vi "Activate Menu.vi"(8 "error in (no error)":errorcluster, 9 "Run mode?":bool, 10 "MenuRef":refnum<k9>, 11 "2D Plot.lvclass in":refnum<class "2D Plot.lvclass">) -> (0 "error out":errorcluster, 3 "2D Plot.lvclass out":refnum<class "2D Plot.lvclass">)   [LabVIEW 2017, in "2D Plot.lvclass"]
uses:
  <vilib>/Math Plots/2D Math Plots/2D Plot/2D Plot/2D Plot.lvclass
  <vilib>/Math Plots/2D Math Plots/2D Plot/2D Plot/2D Plot.lvclass/2D Plot.ctl
panel:
  in  "New Item Names":string="Auto Size Plot Legend"
  in  "Run-time Menu":T1(array[cluster])=[{"menu tag"="", "items to delete"=["APP_SC_CLEAR_GRAPH", "APP_SC_AUTOSCALE_X", "APP_SC_AUTOSCALE_Y", "APP_SC_SMOOTH_UPDATES", "APP_SC_OPTIONAL_PLANE", "APP_SC_SHOW_DIAGRAM"], "new menu"=[{"item names"="Clear Graph", "item tags"="USER_SC_CLEAR_GRAPH", "after item"="APP_SC_CLEAR_GRAPH"}, {"item names"="Autoscale X", "item tags"="USER_SC_AUTOSCALE_X", "after item"="APP_SC_AUTOSCALE_X"}, {"item names"="Autoscale Y", "item tags"="USER_SC_AUTOSCALE_Y", "after item"="USER_SC_AUTOSCALE_X"}], "root?"=TRUE}, {"menu tag"="APP_SC_VISIBLE_ITEMS", "items to delete"=["APP_SC_PLOT_LEGEND", "APP_SC_SCALE_LEGEND", "APP_SC_GRAPH_PALETTE", "APP_SC_CURSOR_LEGEND", "APP_SC_X_SCROLLBAR", "APP_SC_X_SCALE", "APP_SC_Y_SCALE", "APP_SC_UNIT_LABEL"], "new menu"=[{"item names"="Plot Legend", "item tags"="USER_SC_PLOT_LEGEND", "after item"="APP_SC_SEPERATOR"}, {"item names"="Scale Legend", "item tags"="USER_SC_SCALE_LEGEND", "after item"="USER_SC_PLOT_LEGEND"}, {"item names"="Graph Palette", "item tags"="USER_SC_GRAPH_PALETTE", "after item"="USER_SC_SCALE_LEGEND"}, {"item names"="Cursor Legend", "item tags"="USER_SC_CURSOR_LEGEND", "after item"="USER_SC_GRAPH_PALETTE"}, {"item names"="X Scrollbar", "item tags"="USER_SC_X_SCROLLBAR", "after item"="USER_SC_CURSOR_LEGEND"}, {"item names"="-", "item tags"="APP_SC_SEPERATOR", "after item"="USER_SC_X_SCROLLBAR"}, {"item names"="X Scale", "item tags"="USER_SC_X_SCALE", "after item"="APP_SC_SEPERATOR"}, {"item names"="Y Scale", "item tags"="USER_SC_Y_SCALE", "after item"="USER_SC_X_SCALE"}], "root?"=FALSE}]
  in  "Edit-time Menu":T1(array[cluster])=[{"menu tag"="", "items to delete"=["APP_SC_AUTOSCALE_X", "APP_SC_AUTOSCALE_Y", "APP_SC_SMOOTH_UPDATES", "APP_SC_OPTIONAL_PLANE", "APP_SC_PROPERTIES"], "new menu"=[{"item names"="Autoscale X", "item tags"="USER_SC_AUTOSCALE_X", "after item"="APP_SC_AUTOSCALE_X"}, {"item names"="Autoscale Y", "item tags"="USER_SC_AUTOSCALE_Y", "after item"="USER_SC_AUTOSCALE_X"}, {"item names"="Properties", "item tags"="USER_SC_PROPERTIES", "after item"="APP_SC_SEPARATOR"}], "root?"=TRUE}, {"menu tag"="APP_SC_VISIBLE_ITEMS", "items to delete"=["APP_SC_PLOT_LEGEND", "APP_SC_SCALE_LEGEND", "APP_SC_GRAPH_PALETTE", "APP_SC_CURSOR_LEGEND", "APP_SC_X_SCROLLBAR", "APP_SC_X_SCALE", "APP_SC_Y_SCALE", "APP_SC_UNIT_LABEL"], "new menu"=[{"item names"="Plot Legend", "item tags"="USER_SC_PLOT_LEGEND", "after item"="APP_SC_SEPERATOR"}, {"item names"="Scale Legend", "item tags"="USER_SC_SCALE_LEGEND", "after item"="USER_SC_PLOT_LEGEND"}, {"item names"="Graph Palette", "item tags"="USER_SC_GRAPH_PALETTE", "after item"="USER_SC_SCALE_LEGEND"}, {"item names"="Cursor Legend", "item tags"="USER_SC_CURSOR_LEGEND", "after item"="USER_SC_GRAPH_PALETTE"}, {"item names"="X Scrollbar", "item tags"="USER_SC_X_SCROLLBAR", "after item"="USER_SC_CURSOR_LEGEND"}, {"item names"="-", "item tags"="APP_SC_SEPERATOR", "after item"="USER_SC_X_SCROLLBAR"}, {"item names"="X Scale", "item tags"="USER_SC_X_SCALE", "after item"="APP_SC_SEPERATOR"}, {"item names"="Y Scale", "item tags"="USER_SC_Y_SCALE", "after item"="USER_SC_X_SCALE"}], "root?"=FALSE}, {"menu tag"="APP_SC_ADVANCED", "items to delete"=["APP_SC_SHOW_DIAGRAM"], "new menu"=[], "root?"=FALSE}]
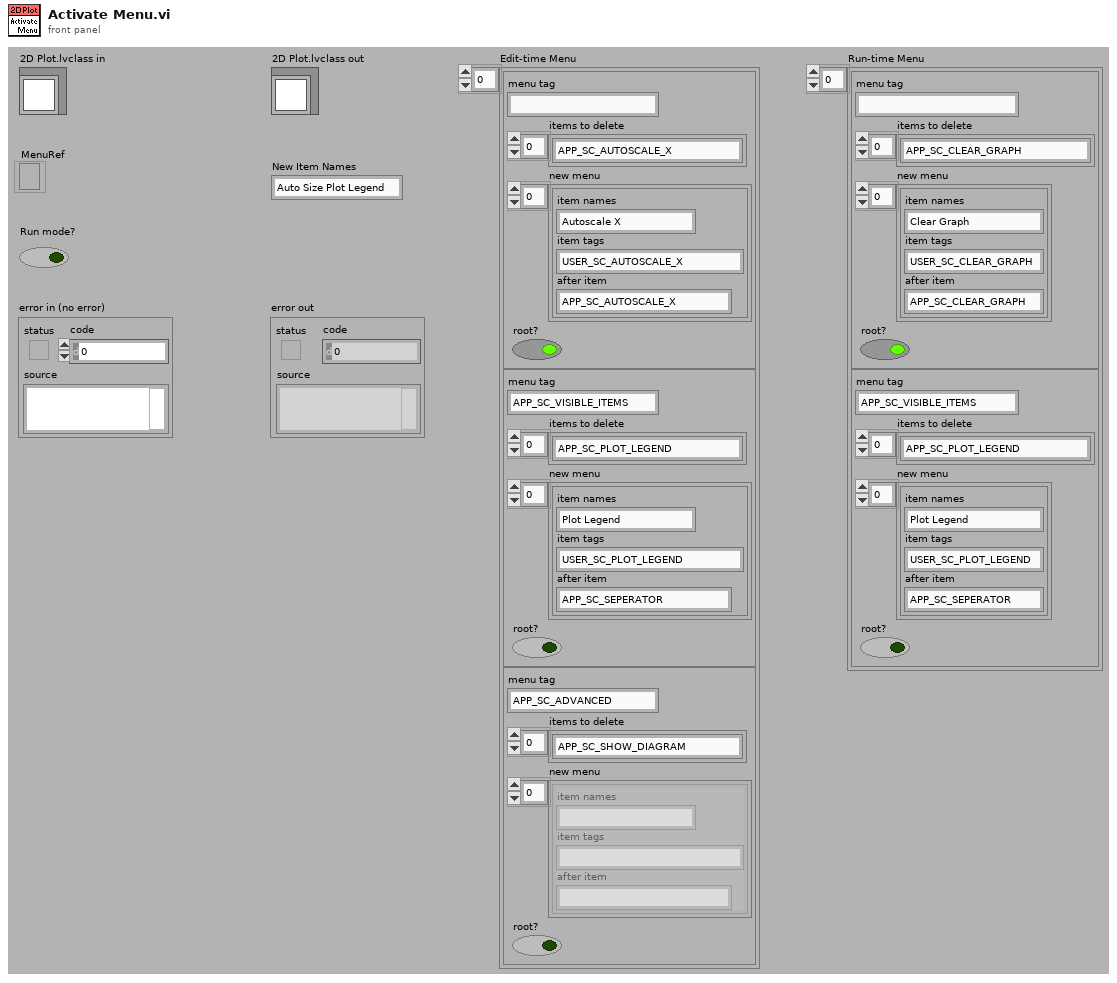
[diagram p1: front panel]
types:
  T1 = cluster{"menu tag":string, "items to delete":string[], "new menu":cluster{"item names":string, "item tags":string, "after item":string}[], "root?":bool}[]
  T2 = typedef "2D Plot.lvclass/Scale Array.ctl" = T3[]
  T3 = typedef "2D Plot.lvclass/Scale Cluster.ctl" = cluster{"General":cluster{"Editable":bool, "Flipped":bool, "Mapping Mode":u8, "Visible":bool, "Style":u8, "Scale Fit":u8}, "Offset and Multiplier":T4, "Range":cluster{"Minimum":dbl, "Maximum":dbl, "Increment":dbl, "Minor Increment":dbl, "Start":dbl}, "Tick Color":cluster{"Major Color":u32, "Minor Color":u32}, "Gird Color":cluster{"Major Color":u32, "Minor Color":u32}, "Marker":cluster{"Visible":bool, "FG Color":u32, "BG Color":u32, "Font Name":string, "Font Size":u32, "Font Bold":bool, "Font Italic":bool, "Font Strikeout":bool, "Font Underline":bool}, "Name Label":cluster{"Visible":bool, "FG Color":u32, "BG Color":u32, "Font Name":string, "Font Size":u32, "Font Bold":bool, "Font Italic":bool, "Font Strikeout":bool, "Font Underline":bool, "Justification":enum16{"Left", "Center", "Right"}, "Text":string}}
  T4 = typedef "LVOffsetAndMultiplierTypeDef.ctl" = cluster{"Offset":dbl, "Multiplier":dbl}
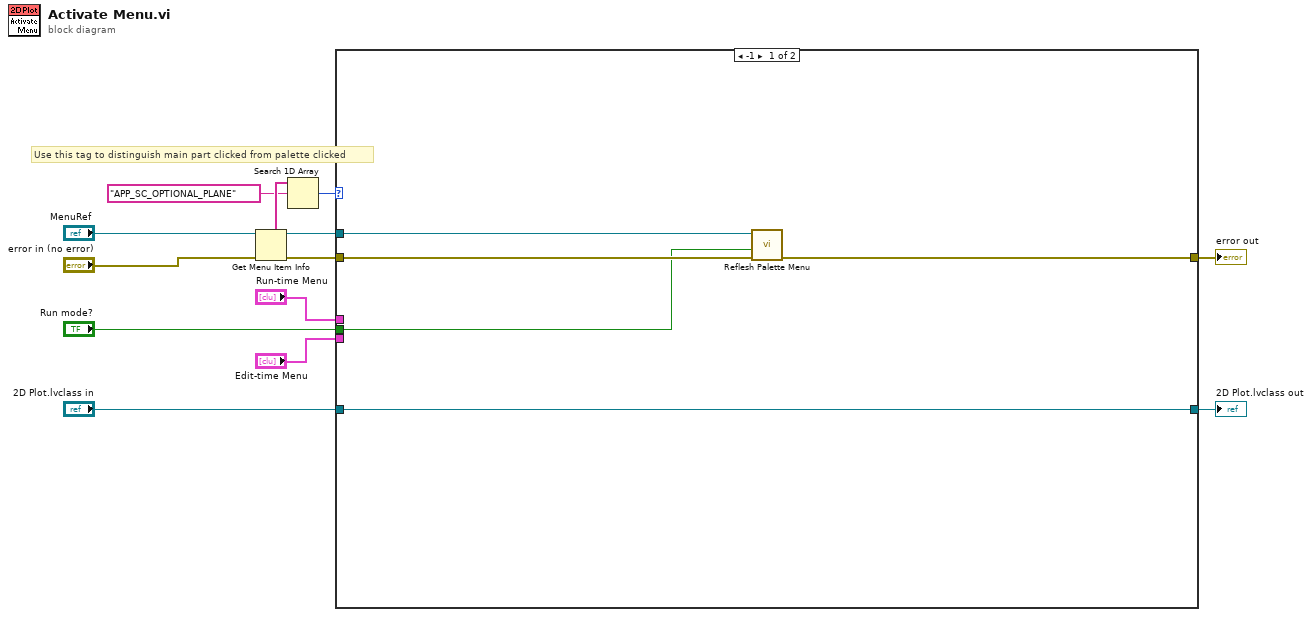
[diagram p0: block diagram]
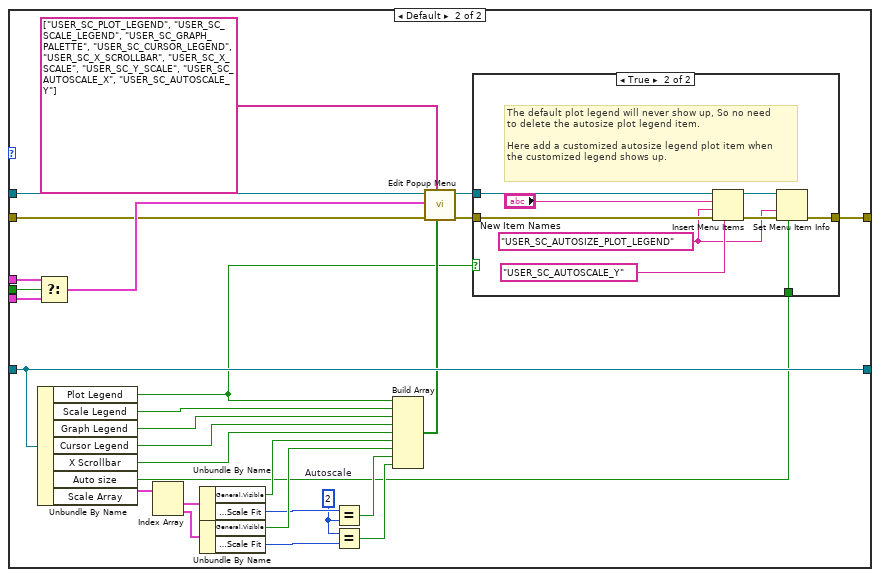
[diagram p2: hidden frame]
diagram:
  # "Use this tag to distinguish main part clicked from palette clicked"
  n1 = Get Menu Item Info(8:"error in (no error)", 11:"MenuRef") -> (0:w7:errorcluster, 3:w11:refnum<k9>, 5:w10:string[])  [unwired: 5 out]
  n2 = Search 1D Array(1D array=w10, element="APP_SC_OPTIONAL_PLANE") -> (index of element=w8:i32)  [unwired: 1 out]
  n3 = case shown="-1" w8 {
    tunnel: "2D Plot.lvclass in" -> [w18 w39]
    tunnel: "Run mode?" -> [w15 w46]
    tunnel: "Run-time Menu" -> [_ w45]
    tunnel: "Edit-time Menu" -> [_ w44]
    tunnel: w11 -> [w17 w43]
    tunnel: w7 -> [w16 w41]
    tunnel: [w14 w21] -> w2
    tunnel: [w18 w39] -> w1
    frame -1 {
      n4 = call <vilib>:"Reflesh Palette Menu.vi"("error in (no error)"=w16, "Run Mode?"=w15, "MenuRef"=w17) -> ("error out"=w14:errorcluster)  [unwired: 8 in]
    }
    frame Default {
      w25 = u8 2  # Autoscale
      n5 = Unbundle By Name(w39) -> ("Plot Legend"=w20:bool, "Scale Legend"=w38:bool, "Graph Legend"=w37:bool, "Cursor Legend"=w36:bool, "X Scrollbar"=w35:bool, "Auto size"=w19:bool, "Scale Array"=w34:T2)
      n6 = Select(t=w45, s=w46, f=w44) -> (s? t:f=w42:T1)
      n7 = Index Array(array=w34) -> (element #1=w33:T3, element #2=w31:T3)  [unwired: 2 in]
      n8 = Unbundle By Name(w33) -> ("General.Visible"=w32:bool, "General.Scale Fit"=w26:u8)
      n9 = Unbundle By Name(w31) -> ("General.Visible"=w30:bool, "General.Scale Fit"=w28:u8)
      n10 = Equal?(x=w26, y=w25) -> (x = y?=w24:bool)
      n11 = Equal?(x=w25, y=w28) -> (x = y?=w27:bool)
      n12 = Build Array(w20, w38, w37, w36, w35, w32, w30, w24, w27) -> (w29:bool[])
      n13 = call <vilib>:"Edit Popup Menu.vi"("User Menu States"=w29, "User Menu Items"=string[] ["USER_SC_PLOT_LEGEND", "USER_SC_SCALE_LEGEND", "USER_SC_GRAPH_PALETTE", "USER_SC_CURSOR_LEGEND", "USER_SC_X_SCROLLBAR", "USER_SC_X_SCALE", "USER_SC_Y_SCALE", "USER_SC_AUTOSCALE_X", "USER_SC_AUTOSCALE_Y"] ("Array"), "error in (no error)"=w41, "Menu Operation Cluster"=w42, "Menu Ref In"=w43) -> ("error out"=w23:errorcluster, "Menu Ref Out"=w22:refnum<k9>)  [unwired: 5 out]
      n14 = case shown="True" w20 {
        tunnel: w22 -> [_ w56]
        tunnel: w23 -> [w47 w53]
        tunnel: [w47 w50] -> w21
        tunnel: w19 -> [_ w48]
        frame False {
        }
        frame True {
          w49 = "USER_SC_AUTOSIZE_PLOT_LEGEND"
          # "The default plot legend will never show up, So no need\nto delete the autosize plot legend item.\n\nHere add a customized autosize legend plot item when\nthe customized legend shows up."
          n15 = Insert Menu Items(4:"USER_SC_AUTOSCALE_Y" ("after item"), 6:w53, 7:w49, 8:"New Item Names", 9:w56) -> (0:w51:errorcluster, 3:w52:refnum<k9>)  [unwired: 2 out]
          n16 = Set Menu Item Info(6:w48, 7:w49, 8:w51, 11:w52) -> (0:w50:errorcluster)  [unwired: 4 out]
        }
      }
    }
  }
  "2D Plot.lvclass out" <- w1
  "error out" <- w2
